vi "Larger video window queue interface.vi"(6 "Function":T3(ring), 7 "Window is open?":bool, 8 "error in (no error)":errorcluster, 10 "Image name":string="Vid 1", 11 "Cam videos cluster in":T4 {"Vid4 Rel time (ms)" format="%.0f ms"; "Vid3 Rel time (ms)" format="%.0f ms"; "Vid2 Rel time (ms)" format="%.0f ms"; "Vid1 Rel time (ms)" format="%.0f ms"}) -> (3 "Output cluster":T1)   [LabVIEW 2013]
uses:
  Typedefs/Cam videos cluster.ctl
  Window position management/Typedefs/Larger windows queues interface cluster.ctl
  Typedefs/Larger window queue ref.ctl
  Typedefs/Larger window queue cluster.ctl
  <vilib>/vision/Image Controls.llb/IMAQ Image.ctl
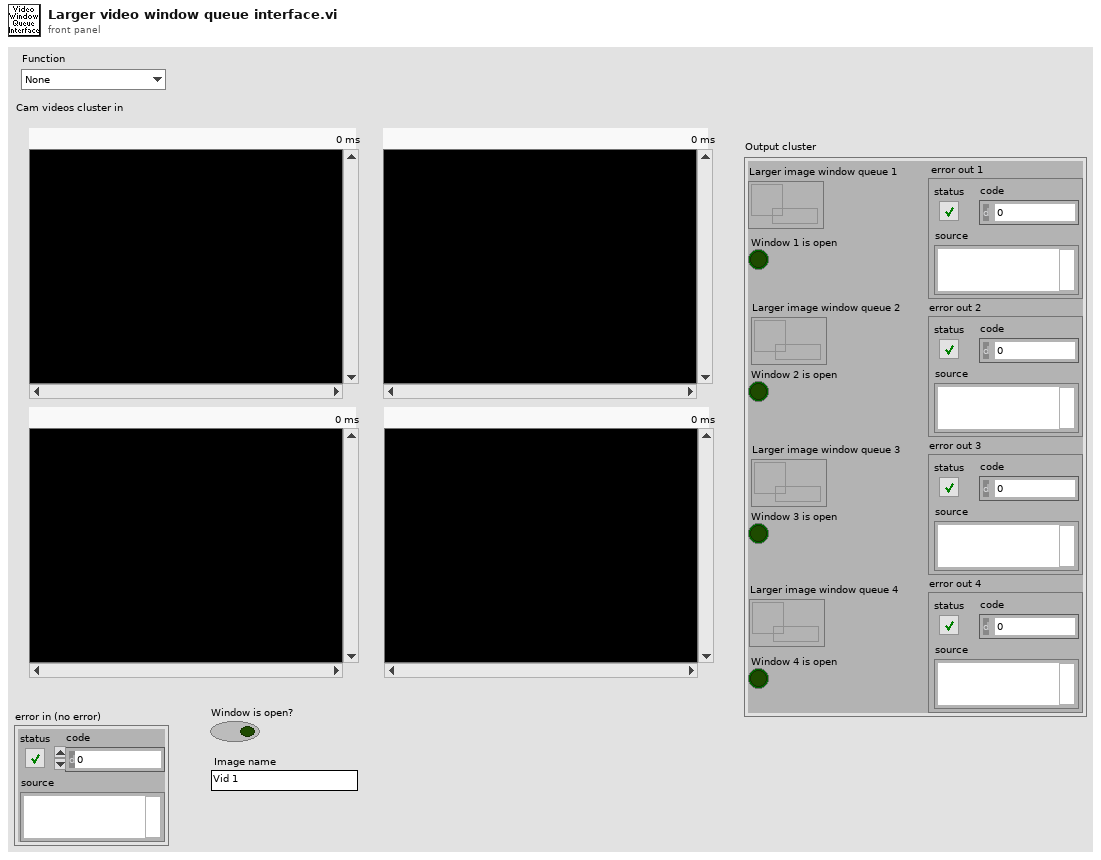
[diagram p1: front panel]
types:
  T1 = typedef "Larger windows queues interface cluster.ctl" = cluster{"error out 1":errorcluster, "Window 1 is open":bool, "error out 2":errorcluster, "Window 2 is open":bool, "error out 3":errorcluster, "Window 3 is open":bool, "error out 4":errorcluster, "Window 4 is open":bool, "Larger image window queue 1":T2, "Larger image window queue 2":T2, "Larger image window queue 3":T2, "Larger image window queue 4":T2}
  T2 = typedef "Larger window queue ref.ctl" = refnum<queue>
  T3 = enum16{"None", "Release queue", "Obtain queue", "Enqueue", "Get status", "Set status"}
  T4 = typedef "Cam videos cluster.ctl" = cluster{"Vid 1":T5, "Vid 2":T5, "Vid 3":T5, "Vid 4":T5, "Vid1 Rel time (ms)":u32, "Vid2 Rel time (ms)":u32, "Vid3 Rel time (ms)":u32, "Vid4 Rel time (ms)":u32}
  T5 = typedef "IMAQ Image.ctl" = refnum<image>
  T6 = typedef "Larger window queue cluster.ctl" = cluster{"Vid":T5, "Rel time (ms)":u32}
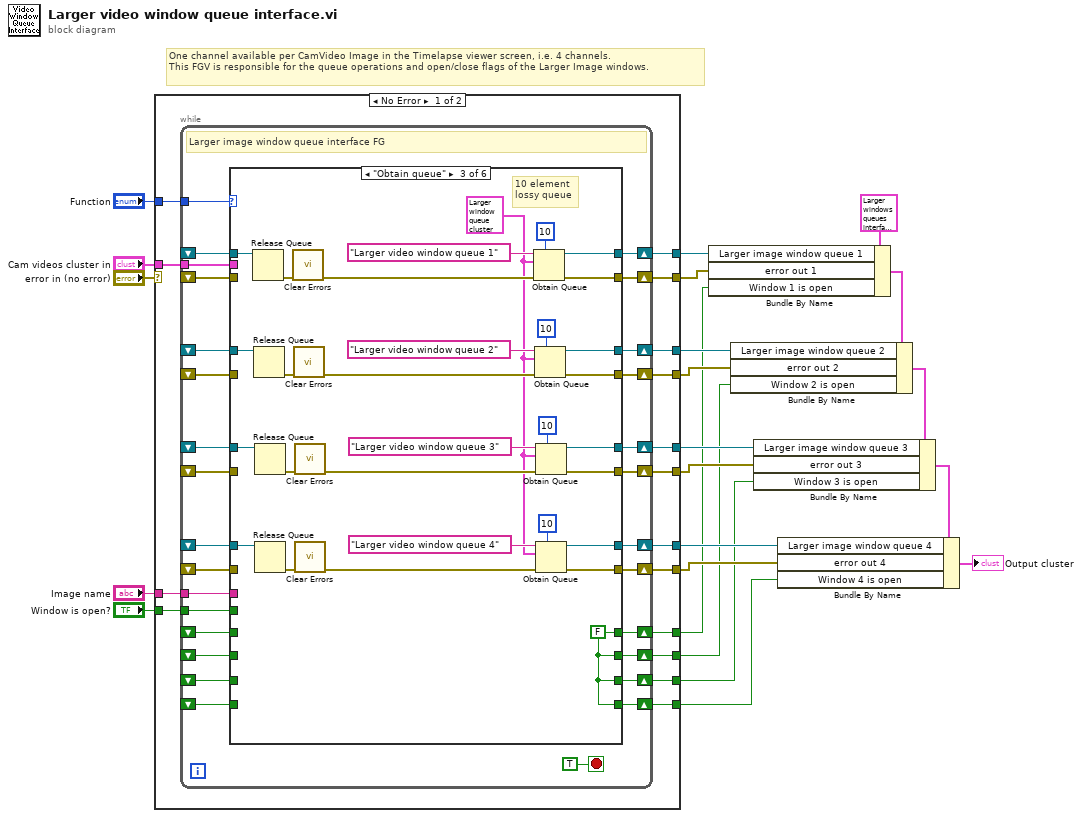
[diagram p0: block diagram]
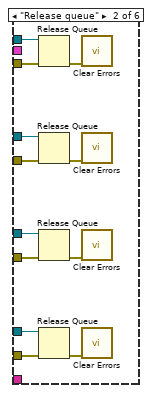
[diagram p3: hidden frame]
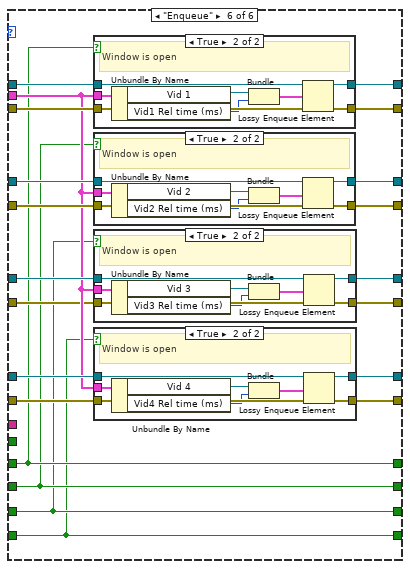
[diagram p10: hidden frame]
diagram:
  # "One channel available per CamVideo Image in the Timelapse viewer screen, i.e. 4 channels.\nThis FGV is responsible for the queue operations and open/close flags of the Larger Image windows."
  n1 = case shown="No Error" "error in (no error)" {
    selector: "error in (no error)" -> [_ w233]
    tunnel: "Function" -> [w38 _]
    tunnel: [w37 _] -> w19
    tunnel: "Cam videos cluster in" -> [w36 _]
    tunnel: [w35 w233] -> w18
    tunnel: [w33 _] -> w9
    tunnel: [w34 _] -> w10
    tunnel: [w32 _] -> w11
    tunnel: [w31 _] -> w12
    tunnel: [w29 _] -> w14
    tunnel: [w30 _] -> w13
    tunnel: [w28 _] -> w6
    tunnel: [w27 _] -> w5
    tunnel: [w26 _] -> w4
    tunnel: [w25 _] -> w3
    tunnel: "Window is open?" -> [w24 _]
    tunnel: "Image name" -> [w23 _]
    frame No Error {
      n2 = while {
        shift-right: [w66] -> w37
        shift-left: _ -> [w64]
        tunnel: w38 -> [w65]
        tunnel: w36 -> [w63]
        shift-right: [w61] -> w35
        shift-left: _ -> [w62]
        shift-right: [w57] -> w33
        shift-left: _ -> [w58]
        shift-right: [w60] -> w34
        shift-left: _ -> [w59]
        shift-right: [w56] -> w32
        shift-left: _ -> [w55]
        shift-right: [w53] -> w31
        shift-left: _ -> [w54]
        shift-right: [w49] -> w29
        shift-left: _ -> [w50]
        shift-right: [w52] -> w30
        shift-left: _ -> [w51]
        shift-right: [w48] -> w28
        shift-left: _ -> [w44]
        shift-right: [w47] -> w27
        shift-left: _ -> [w43]
        shift-right: [w46] -> w26
        shift-left: _ -> [w42]
        shift-right: [w45] -> w25
        shift-left: _ -> [w41]
        tunnel: w24 -> [w40]
        tunnel: w23 -> [w39]
        stop <- TRUE stop-if-true
        # "Larger image window queue interface FG"
        n3 = case shown="\"Obtain queue\"" w65 {
          tunnel: w64 -> [w79 w90 w121 w133 w151 w191]
          tunnel: [w79 _ w118 w133 w151 w192] -> w66
          tunnel: [w72 _ w116 w132 w150 w189] -> w61
          tunnel: w63 -> [_ _ _ _ _ w178]
          tunnel: w62 -> [w72 w89 _ w132 w150 w190]
          tunnel: w58 -> [w78 w80 w108 w131 w149 w182]
          tunnel: [w78 _ w111 w131 w149 w184] -> w57
          tunnel: [w73 _ w113 w130 w148 w183] -> w60
          tunnel: w59 -> [w73 w81 _ w130 w148 w181]
          tunnel: w55 -> [w77 w83 w107 w129 w147 w180]
          tunnel: [w77 _ w104 w129 w147 w185] -> w56
          tunnel: [w74 _ w102 w128 w146 w186] -> w53
          tunnel: w54 -> [w74 w82 _ w128 w146 w176]
          tunnel: w50 -> [w76 w85 w94 w127 w145 w179]
          tunnel: [w76 _ w97 w127 w145 w188] -> w49
          tunnel: [w75 _ w99 w126 w144 w187] -> w52
          tunnel: w51 -> [w75 w84 _ w126 w144 w177]
          tunnel: [w71 _ w92 w125 w137 w175] -> w48
          tunnel: [w70 _ w92 w124 w136 w174] -> w47
          tunnel: [w69 _ w92 w123 w135 w173] -> w46
          tunnel: [w68 _ w92 w122 w134 w172] -> w45
          tunnel: w44 -> [w71 _ _ w125 w141 w175]
          tunnel: w43 -> [w70 _ _ w124 w140 w174]
          tunnel: w42 -> [w69 _ _ w123 w139 w173]
          tunnel: w41 -> [w68 _ _ w122 w138 w172]
          tunnel: w40 -> [_ _ _ _ w142 _]
          tunnel: w39 -> [_ _ _ _ w143 _]
          frame "None", Default {
          }
          frame "Release queue" {
            n4 = Release Queue(queue=w90, error in (no error)=w89) -> (error out=w91:errorcluster)  [unwired: 1 in, 2 out]
            n5 = Release Queue(queue=w80, error in (no error)=w81) -> (error out=w88:errorcluster)  [unwired: 1 in, 2 out]
            n6 = Release Queue(queue=w83, error in (no error)=w82) -> (error out=w87:errorcluster)  [unwired: 1 in, 2 out]
            n7 = Release Queue(queue=w85, error in (no error)=w84) -> (error out=w86:errorcluster)  [unwired: 1 in, 2 out]
            n8 = call <vilib>:"Clear Errors.vi"("error in (no error)"=w91) -> ()  [unwired: 6 in, 1 out]
            n9 = call <vilib>:"Clear Errors.vi"("error in (no error)"=w88) -> ()  [unwired: 6 in, 1 out]
            n10 = call <vilib>:"Clear Errors.vi"("error in (no error)"=w87) -> ()  [unwired: 6 in, 1 out]
            n11 = call <vilib>:"Clear Errors.vi"("error in (no error)"=w86) -> ()  [unwired: 6 in, 1 out]
          }
          frame "Obtain queue" {
            w92 = FALSE ("Window is open?")
            w93 = T6 {"Vid"=refnum, "Rel time (ms)"=0} ("output cluster")
            # "10 element\nlossy queue"
            n12 = Release Queue(queue=w121) -> (error out=w120:errorcluster)  [unwired: 2 in, 2 out]
            n13 = Release Queue(queue=w108) -> (error out=w109:errorcluster)  [unwired: 2 in, 2 out]
            n14 = Release Queue(queue=w107) -> (error out=w106:errorcluster)  [unwired: 2 in, 2 out]
            n15 = Release Queue(queue=w94) -> (error out=w95:errorcluster)  [unwired: 2 in, 2 out]
            n16 = call <vilib>:"Clear Errors.vi"("error in (no error)"=w120) -> ("error out"=w117:errorcluster)  [unwired: 6 in]
            n17 = call <vilib>:"Clear Errors.vi"("error in (no error)"=w109) -> ("error out"=w112:errorcluster)  [unwired: 6 in]
            n18 = call <vilib>:"Clear Errors.vi"("error in (no error)"=w106) -> ("error out"=w103:errorcluster)  [unwired: 6 in]
            n19 = call <vilib>:"Clear Errors.vi"("error in (no error)"=w95) -> ("error out"=w98:errorcluster)  [unwired: 6 in]
            n20 = Obtain Queue(max queue size (-1, unlimited)=10, name (unnamed)="Larger video window queue 1", element data type=w93, error in (no error)=w117) -> (queue out=w118:refnum<queue>, error out=w116:errorcluster)  [unwired: 1 in, 1 out]
            n21 = Obtain Queue(max queue size (-1, unlimited)=10, name (unnamed)="Larger video window queue 2", element data type=w93, error in (no error)=w112) -> (queue out=w111:refnum<queue>, error out=w113:errorcluster)  [unwired: 1 in, 1 out]
            n22 = Obtain Queue(max queue size (-1, unlimited)=10, name (unnamed)="Larger video window queue 3", element data type=w93, error in (no error)=w103) -> (queue out=w104:refnum<queue>, error out=w102:errorcluster)  [unwired: 1 in, 1 out]
            n23 = Obtain Queue(max queue size (-1, unlimited)=10, name (unnamed)="Larger video window queue 4", element data type=w93, error in (no error)=w98) -> (queue out=w97:refnum<queue>, error out=w99:errorcluster)  [unwired: 1 in, 1 out]
          }
          frame "Get status" {
          }
          frame "Set status" {
            n24 = case shown="Default" w143 {
              tunnel: w142 -> [_ w159 w163 w167 w171]
              tunnel: w141 -> [w155 _ w162 w166 w170]
              tunnel: w140 -> [w154 w158 _ w165 w169]
              tunnel: w139 -> [w153 w157 w161 _ w168]
              tunnel: w138 -> [w152 w156 w160 w164 _]
              tunnel: [w155 w159 w162 w166 w170] -> w137
              tunnel: [w154 w158 w163 w165 w169] -> w136
              tunnel: [w153 w157 w161 w167 w168] -> w135
              tunnel: [w152 w156 w160 w164 w171] -> w134
              frame Default {
              }
              frame "Vid 1" {
              }
              frame "Vid 2" {
              }
              frame "Vid 3" {
              }
              frame "Vid 4" {
              }
            }
          }
          frame "Enqueue" {
            n25 = case shown="True" w175 {
              tunnel: w178 -> [_ w228]
              tunnel: w191 -> [w224 w232]
              tunnel: [w223 w231] -> w189
              tunnel: [w224 w230] -> w192
              tunnel: w190 -> [w223 w229]
              frame False {
                # "Window is not open"
              }
              frame True {
                # "Window is open"
                n26 = Unbundle By Name(w228) -> ("Vid 1"=w226:T5, "Vid1 Rel time (ms)"=w227:u32)
                n27 = Bundle("Vid 1"=w226, "Vid1 Rel time (ms)"=w227) -> (w225:cluster{"Vid 1":T5, "Vid1 Rel time (ms)":u32})  [unwired: 1 in]
                n28 = Lossy Enqueue Element(queue=w232, element=w225, error in (no error)=w229) -> (queue out=w230:refnum<queue>, error out=w231:errorcluster)  [unwired: 2 out]
              }
            }
            n29 = case shown="True" w174 {
              tunnel: w178 -> [_ w218]
              tunnel: w182 -> [w214 w222]
              tunnel: [w213 w221] -> w183
              tunnel: [w214 w220] -> w184
              tunnel: w181 -> [w213 w219]
              frame False {
                # "Window is not open"
              }
              frame True {
                # "Window is open"
                n30 = Unbundle By Name(w218) -> ("Vid 2"=w217:T5, "Vid2 Rel time (ms)"=w216:u32)
                n31 = Bundle("Vid 2"=w217, "Vid2 Rel time (ms)"=w216) -> (w215:cluster{"Vid 2":T5, "Vid2 Rel time (ms)":u32})  [unwired: 1 in]
                n32 = Lossy Enqueue Element(queue=w222, element=w215, error in (no error)=w219) -> (queue out=w220:refnum<queue>, error out=w221:errorcluster)  [unwired: 2 out]
              }
            }
            n33 = case shown="True" w173 {
              tunnel: w178 -> [_ w208]
              tunnel: w180 -> [w204 w212]
              tunnel: [w203 w211] -> w186
              tunnel: [w204 w210] -> w185
              tunnel: w176 -> [w203 w209]
              frame False {
                # "Window is not open"
              }
              frame True {
                # "Window is open"
                n34 = Unbundle By Name(w208) -> ("Vid 3"=w207:T5, "Vid3 Rel time (ms)"=w206:u32)
                n35 = Bundle("Vid 3"=w207, "Vid3 Rel time (ms)"=w206) -> (w205:cluster{"Vid 3":T5, "Vid3 Rel time (ms)":u32})  [unwired: 1 in]
                n36 = Lossy Enqueue Element(queue=w212, element=w205, error in (no error)=w209) -> (queue out=w210:refnum<queue>, error out=w211:errorcluster)  [unwired: 2 out]
              }
            }
            n37 = case shown="True" w172 {
              tunnel: w178 -> [_ w198]
              tunnel: w179 -> [w194 w202]
              tunnel: [w193 w201] -> w187
              tunnel: [w194 w200] -> w188
              tunnel: w177 -> [w193 w199]
              frame False {
                # "Window is not open"
              }
              frame True {
                # "Window is open"
                n38 = Unbundle By Name(w198) -> ("Vid 4"=w197:T5, "Vid4 Rel time (ms)"=w196:u32)
                n39 = Bundle("Vid 4"=w197, "Vid4 Rel time (ms)"=w196) -> (w195:cluster{"Vid 4":T5, "Vid4 Rel time (ms)":u32})  [unwired: 1 in]
                n40 = Lossy Enqueue Element(queue=w202, element=w195, error in (no error)=w199) -> (queue out=w200:refnum<queue>, error out=w201:errorcluster)  [unwired: 2 out]
              }
            }
          }
        }
      }
    }
    frame Error {
    }
  }
  n41 = Bundle By Name(cluster=T1 {"error out 1"={"status"=FALSE, "code"=0, "source"=""}, "Window 1 is open"=FALSE, "error out 2"={"status"=FALSE, "code"=0, "source"=""}, "Window 2 is open"=FALSE, "error out 3"={"status"=FALSE, "code"=0, "source"=""}, "Window 3 is open"=FALSE, "error out 4"={"status"=FALSE, "code"=0, "source"=""}, "Window 4 is open"=FALSE, "Larger image window queue 1"=refnum, "Larger image window queue 2"=refnum, "Larger image window queue 3"=refnum, "Larger image window queue 4"=refnum} ("Output cluster"), "Larger image window queue 1"=w19, "error out 1"=w18, "Window 1 is open"=w6) -> (w17:T1)
  n42 = Bundle By Name(cluster=w17, "Larger image window queue 2"=w9, "error out 2"=w10, "Window 2 is open"=w5) -> (w16:T1)
  n43 = Bundle By Name(cluster=w16, "Larger image window queue 3"=w11, "error out 3"=w12, "Window 3 is open"=w4) -> (w15:T1)
  n44 = Bundle By Name(cluster=w15, "Larger image window queue 4"=w14, "error out 4"=w13, "Window 4 is open"=w3) -> (→"Output cluster":T1)
